vi "Check Parameter.vi"(6 "Options in":T1={"DbType"=-1, "Direction"=-1, "Size"=-1, "Precision"=255, "Scale"=255} {"Direction" items=["Input"=1, "Output"=2, "InputOutput"=3, "ReturnValue"=6]; "DbType" items=["AnsiString"=0, "Binary"=1, "Byte"=2, "Boolean"=3, "Currency"=4, "Date"=5, "DateTime"=6, "Decimal"=7, "Double"=8, "Guid"=9, "Int16"=10, "Int32"=11, "Int64"=12, "Object"=13, "SByte"=14, "Single"=15, "String"=16, "Time"=17, "UInt16"=18, "UInt32"=19, "UInt64"=20, "VarNumeric"=21, "AnsiStringFixedLength"=22, "StringFixedLength"=23, "Xml"=25, "DateTime2"=26, "DateTimeOffset"=27]}, 8 "error in (no error)":errorcluster, 9 "value in":variant, 10 "name in":string, 11 "ODBCConnection in":refnum<class "DBC.lvclass">) -> (0 "error out":errorcluster, 1 "value out":variant, 2 "name out":string, 3 "ODBCConnection out":refnum<class "DBC.lvclass">, 4 "Options out":T1={"DbType"=-1, "Direction"=-1, "Size"=-1, "Precision"=255, "Scale"=255} {"Direction" items=["Input"=1, "Output"=2, "InputOutput"=3, "ReturnValue"=6]; "DbType" items=["AnsiString"=0, "Binary"=1, "Byte"=2, "Boolean"=3, "Currency"=4, "Date"=5, "DateTime"=6, "Decimal"=7, "Double"=8, "Guid"=9, "Int16"=10, "Int32"=11, "Int64"=12, "Object"=13, "SByte"=14, "Single"=15, "String"=16, "Time"=17, "UInt16"=18, "UInt32"=19, "UInt64"=20, "VarNumeric"=21, "AnsiStringFixedLength"=22, "StringFixedLength"=23, "Xml"=25, "DateTime2"=26, "DateTimeOffset"=27]})   [LabVIEW 2020, in "ORM_DBC_Odbc.lvlib" / "DBC.lvclass"]
uses:
  DBC.lvclass
  <vilib>/Viviota/shared/ORM_DBC_dotNet.lvlibp/dbcDotNet/ORM_DBC_dotNet.lvclass
  <vilib>/Utility/Data Type/NI_Data Type.lvlib
  <vilib>/JDP Science/JSONtext/JSONtext.lvlib
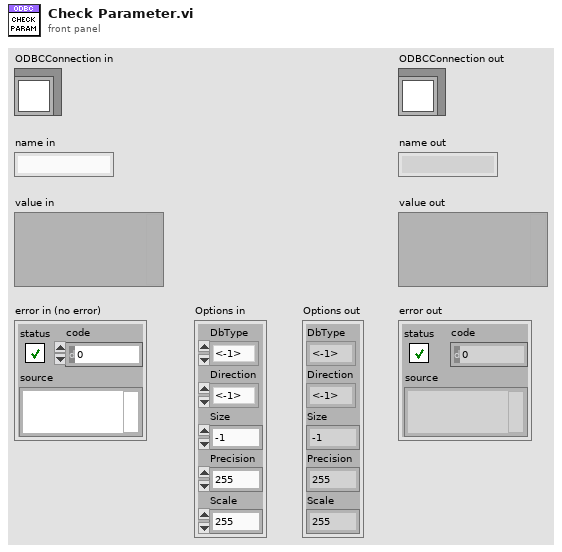
[diagram p1: front panel]
types:
  T1 = cluster{"DbType":i32, "Direction":i32, "Size":i32, "Precision":u8, "Scale":u8}
  T2 = typedef "NI_Data Type.lvlib/Data Type.ctl" = enum8{"Invalid Type", "Void", "I8", "I16", "I32", "I64", "U8", "U16", "U32", "U64", "Single Float", "Double Float", "Extended Float", "Single Complex", "Double Complex", "Extended Complex", "Enum U8", "Enum U16", "Enum U32", "Enum U64", "Single Float With Unit", "Double Float With Unit", "Extended Float With Unit", "Single Complex with Unit", "Double Complex with Unit", "Extended Complex with Unit", "Boolean", "String", "Path", "Picture", "Tag", "Array", "Cluster", "Variant", "LV Variant", "Waveform", "Timestamp", "Digital Waveform", "Digital Data", "ExpressData", "Refnum", "External Data", "VI", "Poly VI", "LabVIEW Class Instance", "Fixed Point", "Set Collection", "Map Collection"}
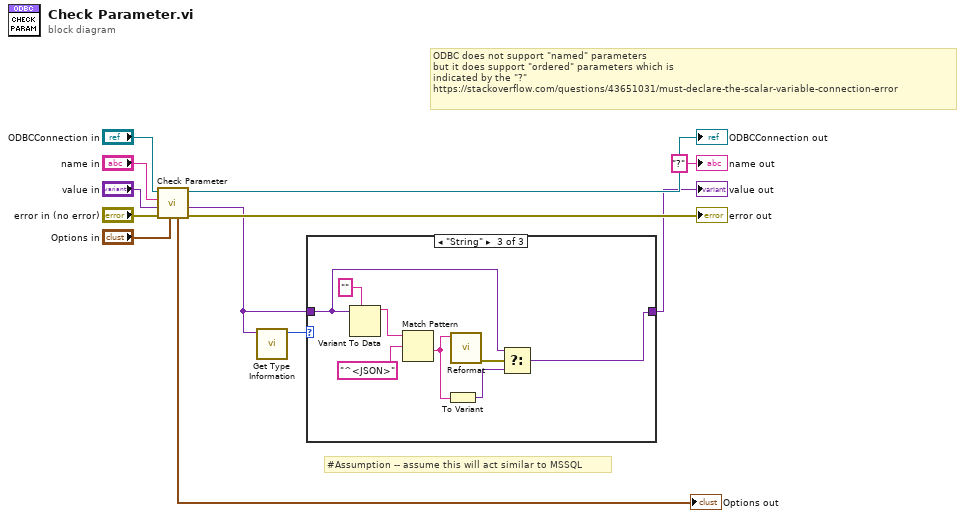
[diagram p0: block diagram]
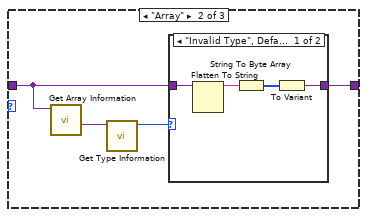
[diagram p3: hidden frame]
diagram:
  # "#Assumption -- assume this will act similar to MSSQL"
  # "ODBC does not support \"named\" parameters\nbut it does support \"ordered\" parameters which is \nindicated by the \"?\"\nhttps://stackoverflow.com/questions/43651031/must-declare-the-scalar-variable-connection-error"
  n1 = call-parent "Check Parameter.vi"("Options in"="Options in", "error in (no error)"="error in (no error)", "value in"="value in", "name in"="name in", "DbConnection in"="ODBCConnection in") -> ("error out"=→"error out":errorcluster, "value out"=w2:variant, "DbConnection out"=→"ODBCConnection out":refnum<class "DBC.lvclass">, "Options out"=→"Options out":T1)  [unwired: 2 in, 1 out]
  n2 = call <vilib>:"Get Type Information.vi"("variant"=w2) -> ("type"=w3:T2)  [unwired: 6 in, 4 out]
  n3 = case shown="\"String\"" w3 {
    tunnel: w2 -> [w13 w16 w24]
    tunnel: [w13 w17 w23] -> w1
    frame "Invalid Type", Default {
    }
    frame "Array" {
      n4 = call <vilib>:"Get Array Information.vi"("variant"=w16) -> ("array element data type"=w15:variant)  [unwired: 7 in, 3 out]
      n5 = call <vilib>:"Get Type Information.vi"("variant"=w15) -> ("type"=w14:T2)  [unwired: 6 in, 4 out]
      n6 = case shown="\"Invalid Type\", Default" w14 {
        tunnel: [w19 w22] -> w17
        tunnel: w16 -> [w18 w22]
        frame "Invalid Type", Default {
          n7 = Flatten To String(anything=w18) -> (data string=w21:string)  [unwired: 3 in, 2 out]
          n8 = String To Byte Array(string=w21) -> (unsigned byte array=w20:u8[])
          n9 = To Variant(anything=w20) -> (Variant=w19:variant)
        }
        frame "U8" {
        }
      }
    }
    frame "String" {
      n10 = Variant To Data(type="", Variant=w24) -> (data=w28:string)  [unwired: 1 in, 1 out]
      n11 = Match Pattern(string=w28, regular expression="^<JSON>") -> (after substring=w25:string)  [unwired: 1 in, 3 out]
      n12 = To Variant(anything=w25) -> (Variant=w26:variant)
      n13 = call <vilib>:"Reformat.vi"("JSON"=w25) -> ("error out"=w27:errorcluster)  [unwired: 7 in, 3 out]
      n14 = Select(t=w24, s=w27, f=w26) -> (s? t:f=w23:variant)
    }
  }
  "value out" <- w1
  "name out" <- "?" ("name out")
